vi "SQLite DB Path.vi"(9 "Password":string, 10 "ping":bool, 11 "database":string="database1.db") -> (3 "Path out":string)   [LabVIEW 2016, in "SQLite Lib.lvlib"]
uses:
  SQLite Lib.lvlib
  <vilib>/Utility/sysdir.llb/System Directory Type.ctl
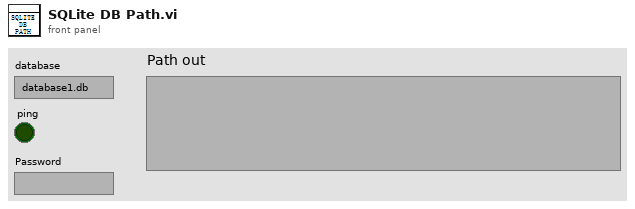
[diagram p1: front panel]
types:
  T1 = typedef "System Directory Type.ctl" = i32
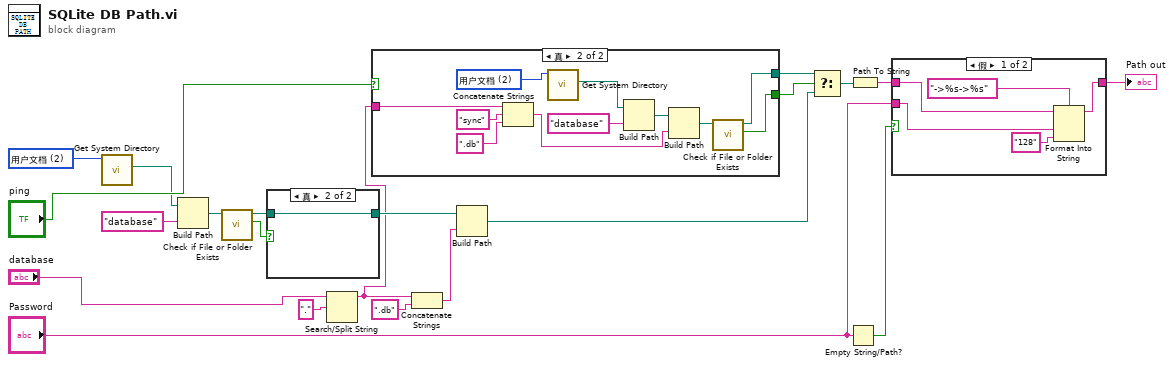
[diagram p0: block diagram]
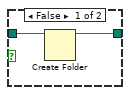
[diagram p2: hidden frame]
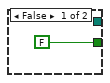
[diagram p3: hidden frame]
diagram:
  w9 = T1 2 items=["用户目录"=0, "用户桌面"=1, "用户文档"=2, "用户应用程序数据"=3, "用户设置"=4, "用户临时目录"=5, "公共文档"=6, "公共应用程序数据"=7, "公共设置"=8, "公共缓存"=13, "系统核心库"=9, "系统安装库"=10, "应用程序文件"=11, "启动盘根目录"=12] ("system directory type")
  n1 = call <vilib>:"Get System Directory.vi"("system directory type"=w9) -> ("system directory"=w8:path)  [unwired: 10 in]
  n2 = Build Path(base path=w8, name or relative path="database" ("名称或相对路径")) -> (appended path=w6:path)
  n3 = call <vilib>:"Check if File or Folder Exists.vi"("path"=w6) -> ("file or folder exists?"=w14:bool, "dup path"=w13:path)  [unwired: 8 in, 1 out]
  n4 = case shown="真" w14 {
    tunnel: w13 -> [w23 w24]
    tunnel: [w22 w24] -> w12
    frame False {
      n5 = Create Folder(path (use dialog)=w23) -> (created path=w22:path)  [unwired: 2 in, 2 out]
    }
    frame True {
    }
  }
  n6 = Search/Split String(string="database", search string/char (-)="." ("搜索字符串/字符(-)")) -> (substring before match=w1:string)  [unwired: 1 in, 2 out]
  n7 = case shown="真" "ping" {
    tunnel: [FALSE ("file or folder exists?") w31] -> w5
    tunnel: [_ w30] -> w4
    tunnel: w1 -> [_ w26]
    frame False {
    }
    frame True {
      w36 = T1 2 items=["用户目录"=0, "用户桌面"=1, "用户文档"=2, "用户应用程序数据"=3, "用户设置"=4, "用户临时目录"=5, "公共文档"=6, "公共应用程序数据"=7, "公共设置"=8, "公共缓存"=13, "系统核心库"=9, "系统安装库"=10, "应用程序文件"=11, "启动盘根目录"=12] ("system directory type")
      n8 = Concatenate Strings(w26, "sync" ("字符串"), ".db" ("字符串")) -> (w27:string)
      n9 = call <vilib>:"Get System Directory.vi"("system directory type"=w36) -> ("system directory"=w35:path)  [unwired: 10 in]
      n10 = Build Path(base path=w35, name or relative path="database" ("名称或相对路径")) -> (appended path=w33:path)
      n11 = Build Path(base path=w33, name or relative path=w27) -> (appended path=w32:path)
      n12 = call <vilib>:"Check if File or Folder Exists.vi"("path"=w32) -> ("file or folder exists?"=w31:bool, "dup path"=w30:path)  [unwired: 8 in, 1 out]
    }
  }
  n13 = Concatenate Strings(w1, ".db" ("字符串")) -> (w11:string)
  n14 = Build Path(base path=w12, name or relative path=w11) -> (appended path=w3:path)
  n15 = Select(t=w4, s=w5, f=w3) -> (s? t:f=w2:path)
  n16 = Empty String/Path?(string/path="Password") -> (empty?=w18:bool)
  n17 = Path To String(path=w2) -> (string=w21:string)
  n18 = case shown="假" w18 {
    tunnel: w21 -> [w40 w42]
    tunnel: [w39 w42] -> w20
    tunnel: "Password" -> [w37 _]
    frame False {
      n19 = Format Into String(format string="->%s->%s", initial string=w40, w37, "128" ("Enter Password")) -> (resulting string=w39:string)  [unwired: 1 in, 1 out]
    }
    frame True {
    }
  }
  "Path out" <- w20
